vi "GE 5565PIORC.DMA.Block.VISA Return Handler.vi"(8 "error in (no error)":errorcluster, 11 "VISA return value":i32) -> (0 "error out":errorcluster)   [LabVIEW 2016, in "GE 5565PIORC.lvclass"]
uses:
  GE 5565PIORC.lvclass
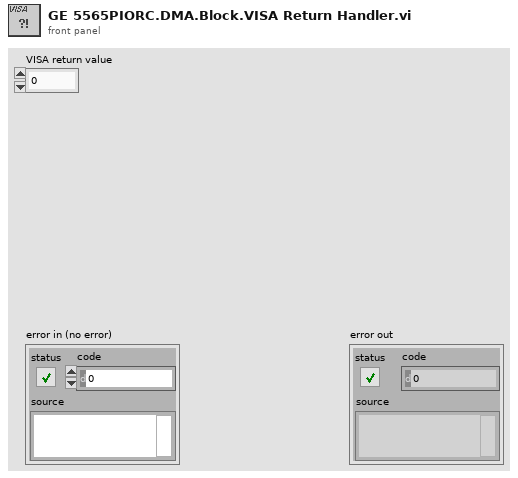
[diagram p1: front panel]
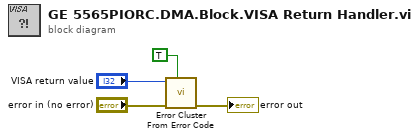
[diagram p0: block diagram]
diagram:
  n1 = call <vilib>:"Error Cluster From Error Code.vi"("show call chain? (False)"=TRUE, "error in (no error)"="error in (no error)", "error code (0)"="VISA return value") -> ("error out"=→"error out":errorcluster)  [unwired: 6 in]
